vi "Core Action.vi"(8 "error in (no error)":errorcluster, 10 "SECS-II Class In":refnum<class "SECS-II Class.lvclass">, 11 "36-List Enabled Alarm Data in":refnum<class "36-List Enabled Alarm Data.lvclass">) -> (0 "error out":errorcluster, 2 "SECS-II Class Out":refnum<class "SECS-II Class.lvclass">, 3 "36-List Enabled Alarm Data out":refnum<class "36-List Enabled Alarm Data.lvclass">)   [LabVIEW 2020, in "SECS Scenarios.lvlib" / "36-List Enabled Alarm Data.lvclass"]
uses:
  36-List Enabled Alarm Data.lvclass
  D:/Dropbox/SECS/SECS_GEM v1.1.0/Com/SECS Scenarios/Scenarios Class/Scenarios Class.lvclass
  SECS Communication/SECS-II Class/SECS-II Class.lvclass
  SECS Communication/S5 Message Class/S5 Message Class.lvclass
  D:/Dropbox/SECS/SECS_GEM v1.1.0/Com/SECS Communication/SECS-II Class/SECS-II Class.lvclass
  Scenarios Class/Reply State.ctl
  Scenarios Class/Scenarios Class.lvclass/Scenarios Class.ctl
  SECS Communication/S5 Message Class/S5F8.ctl
  Scenarios Class/Write Reply State.vi
  Scenarios Class/Read HSMS Class.vi
  SECS Communication/SECS Data Class/Get All ALID Data.vi
  SECS Communication/HSMS Class/HSMS Class.lvclass
  Scenarios Class/Scenarios Class.lvclass
  SECS Communication/SECS Data Class/SECS Data Class.lvclass
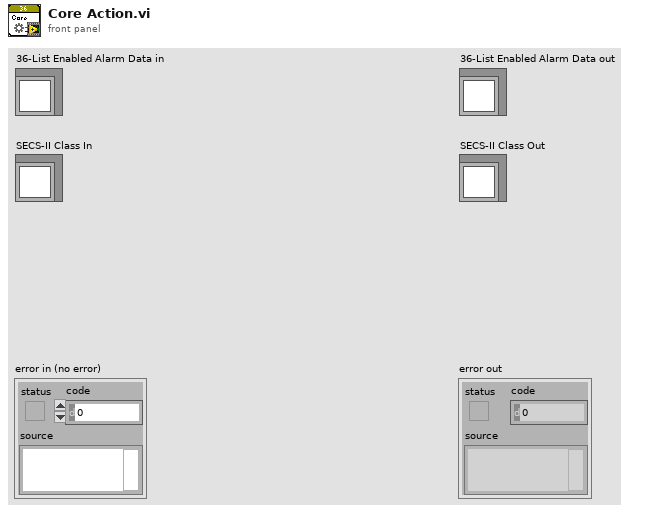
[diagram p1: front panel]
types:
  T1 = typedef "SECS Scenarios.lvlib/Scenarios Class.lvclass/Reply State.ctl" = enum16{"OK", "Illegal Data", "Unknown Stream", "Unknown Function", "Off-Line", "T3 Timeout", "Inner-Timeout"}
  T2 = typedef "SECS Communication.lvlib/S5 Message Class.lvclass/S5F8.ctl" = cluster{"ALCD(Bit8)":bool, "ALID":u32, "ALTX":string}
  T3 = typedef "SECS Communication.lvlib/SECS Data Class.lvclass/ALID Data.ctl" = cluster{"Enable":bool, "ALID":u32, "Name":string, "Description":string, "Source":string, "Status":enum16{"Null", "Normal", "Abnormal", "Warning"}}
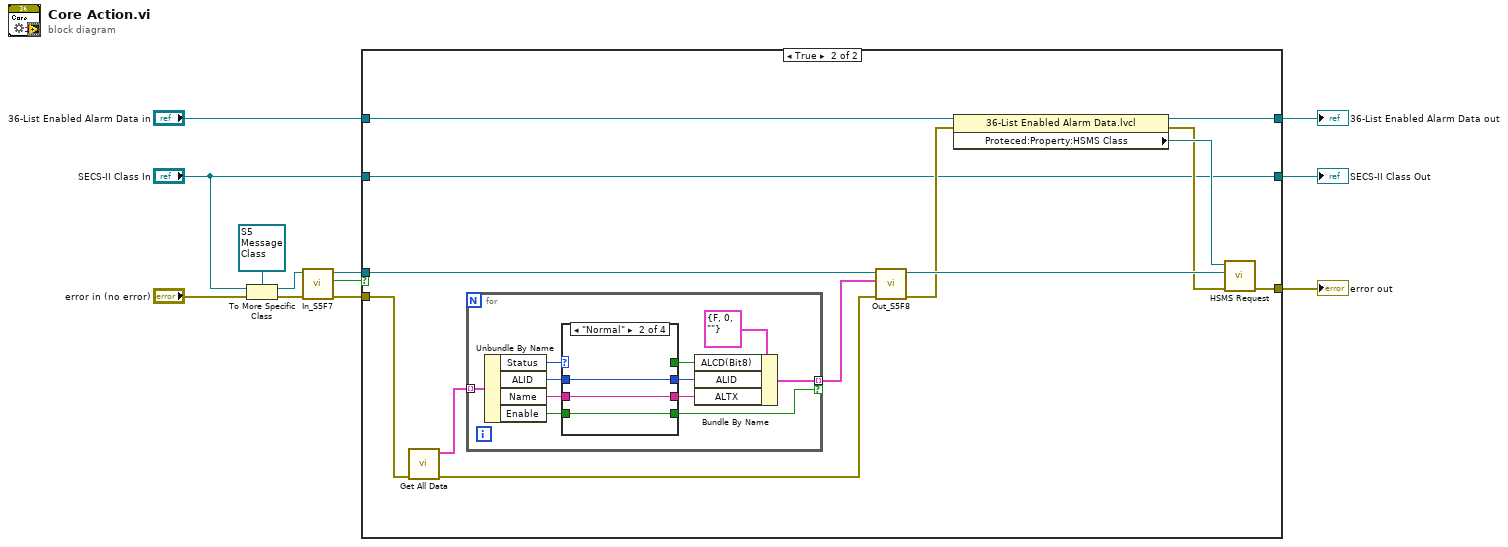
[diagram p0: block diagram]
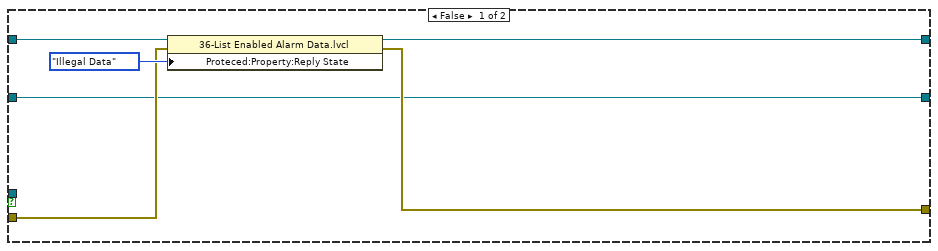
[diagram p2: hidden frame]
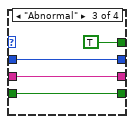
[diagram p4: hidden frame]
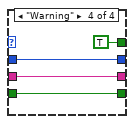
[diagram p5: hidden frame]
diagram:
  n1 = To More Specific Class(target class=refnum<class "S5 Message Class.lvclass"> refnum ("SECS Communication.lvlib:S5 Message Class.lvclass"), reference="SECS-II Class In", error in="error in (no error)") -> (specific class reference=w10:refnum<class "S5 Message Class.lvclass">, error out=w11:errorcluster)
  n2 = call "In_S5F7.vi"("error in (no error)"=w11, "S5 Message Class in"=w10) -> ("error out"=w9:errorcluster, "Empty?"=w4:bool, "S5 Message Class out"=w8:refnum<class "S5 Message Class.lvclass">)  [unwired: 7 in]
  n3 = case shown="True" w4 {
    tunnel: "36-List Enabled Alarm Data in" -> [w18 w31]
    tunnel: [w17 w30] -> w3
    tunnel: w9 -> [w15 w28]
    tunnel: w8 -> [_ w26]
    tunnel: [w14 w21] -> w1
    tunnel: "SECS-II Class In" -> [w13 w20]
    tunnel: [w13 w20] -> w2
    frame False {
      n4 = property class="36-List Enabled Alarm Data.lvcl"(reference=w18, error in=w15, "Proteced:Property:Reply State"=Reply_State."Illegal Data" ("Reply State")) -> (reference out=w17:refnum<class "36-List Enabled Alarm Data.lvclass">, error out=w14:errorcluster)
    }
    frame True {
      n5 = call-poly "Get All Data.vi"("error in (no error)"=w28) -> ("error out"=w25:errorcluster, "ALID Data"=w27:T3[])  [unwired: 9 in]
      n6 = for {
        tunnel: w27 -> [w38] mode=indexing
        tunnel: [w42] -> w19 mode=indexing if=w32
        n7 = Unbundle By Name(w38) -> ("Status"=w41:enum16{"Null", "Normal", "Abnormal", "Warning"}, "ALID"=w40:u32, "Name"=w39:string, "Enable"=w33:bool)
        n8 = case shown="\"Normal\"" w41 {
          tunnel: w40 -> [w45 w47 w51 w55]
          tunnel: w39 -> [w44 w48 w52 w56]
          tunnel: [w44 w48 w52 w56] -> w35
          tunnel: [w45 w47 w51 w55] -> w36
          tunnel: [_ _ TRUE TRUE] -> w37
          tunnel: w33 -> [w43 w46 w49 w53]
          tunnel: [w43 w46 w49 w53] -> w32
          frame "Null", Default {
          }
          frame "Normal" {
          }
          frame "Abnormal" {
          }
          frame "Warning" {
          }
        }
        n9 = Bundle By Name(cluster=T2 {"ALCD(Bit8)"=FALSE, "ALID"=0, "ALTX"=""} ("S5F8"), "ALCD(Bit8)"=w37, "ALID"=w36, "ALTX"=w35) -> (w42:T2)
      }
      n10 = call "Out_S5F8.vi"("error in (no error)"=w25, "S5F8"=w19, "S5 Message Class in"=w26) -> ("error out"=w23:errorcluster, "S5 Message Class out"=w24:refnum<class "S5 Message Class.lvclass">)  [unwired: 7 in]
      n11 = property class="36-List Enabled Alarm Data.lvcl"(reference=w31, error in=w23) -> (reference out=w30:refnum<class "36-List Enabled Alarm Data.lvclass">, error out=w22:errorcluster, "Proteced:Property:HSMS Class"=w29:refnum<class "HSMS Class.lvclass">)
      n12 = call "HSMS Request.vi"("error in (no error)"=w22, "SECS-II Class In"=w24, "HSMS Class in"=w29) -> ("error out"=w21:errorcluster)  [unwired: 7 in, 1 out]
    }
  }
  "error out" <- w1
  "36-List Enabled Alarm Data out" <- w3
  "SECS-II Class Out" <- w2
